vi "载荷控制.vi"() -> ()   [LabVIEW 2020]
doc: "The Basic Serial Read and Write example performs a Serial Port Read, a Serial Port Write, or a combination of these actions. The user selects the actions (read or write) on the front panel. If both are selected, the VI will write the data first, read data, and then close the VISA session that is opened to the port. This VI will wait until the specified number of bytes is received at the port. Only the number of bytes specified will be read.\n\nINSTRUCTIONS:\n1) Select the serial resource and configuration parameters (baud rate, data bits, parity, stop bits, flow control).\n2) Select the operations to be performed. \n3) Connect the serial port to your device. If no device is available, perform a loopback test by doing one of the following. Short pins 2 and 3 on a RS-232 cable or short pin 4 to pin 8 and pin 5 to pin 9 on a RS-485/422 cable. \n4) Run the VI to see the data read. (The \"read string\" will match the \"string to write\" if a loopback test was performed.)\n\nNote: The parameters set for the serial port must match the parameters of the connected instrument or device. In this example, the bytes to read parameter specifies the number of bytes that the serial port reads. If there were more bytes at the port than the number specified in bytes to read, those bytes would not be read. Also, if you specify to read more bytes than the number of bytes actually read, you might receive a timeout error message.\n\nOn the block diagram, the Configure Serial Port VI sets the configuration parameters. The front panel displays the controls used to configure the basic parameters, such as baud rate, data bits, and parity. Constants configure the other parameters the user probably does not need set. After the VISA Configure Serial Port VI opens the VISA session and configures the port, the VI passes the VISA resource name to other VIs that perform operations on that VISA resource. The VISA Write function sends a command to the serial device and the VISA Read function returns data based on the command. The VISA Close function then closes the reference to the serial device. It is important to close the reference; otherwise communication through with that port through protocols other than VISA might not be possible."
uses:
  <vilib>/Analysis/baseanly.llb/Mean (DBL).vi
  <vilib>/Instr/_visa.llb/VISA Configure Serial Port (Instr).vi
  <vilib>/addons/control/pid/pid.llb/PID (DBL).vi
  <vilib>/Analysis/NI_AALBase.lvlib
  <vilib>/addons/control/pid/NI_PID_pid.lvlib
panel:
  in  "点火/退出":bool
  in  "气缸":dbl
  in  "点火":dbl
  in  "停止3":bool
  out "位移(um）":dbl format="%#.2f"
  out "数据":dbl
  out "原始载荷":dbl format="%#.2f"
  out "当前次数":i32
  in  "选项卡控件":enum32{"设置", "手动", "自动", "循环加载"}(tab)
  in  "温度文件":path
  in  "设置串口":refnum<visa-resource-name>="COM1"
  in  "载荷测量":tag="cDAQ9184-1ADFF13Mod3"
  in  "气流控制":tag="Dev2"
  in  "?":bool
  in  "?":bool
  in  "?":bool
  in  "?":bool
  in  "位置清零":bool
  in  "载荷清零":bool
  in  "开始":bool
  in  "加载":bool
  in  "比例系数":i32 min=0 max=1000
  in  "设定载荷":i32 min=0 max=1000
  in  "形变速率（微米/秒）":i32 min=0
  in  "冷却控制":dbl
  in  "设定温度值 ℃":dbl(slide)=43.790849673202615 scale=0.0..3000.0
  out "MV：":dbl(slide)=18.78965245852964 scale=0.0..6.0
  in  "PID增益":T1={"比例增益(Kc)"=20.0, "积分时间（Ti，分）"=0.008, "微分时间（Td，分）"=0.001} {"微分时间（Td，分）" format="%.3f"; "积分时间（Ti，分）" format="%.3f"; "比例增益(Kc)" format="%.3f"}
  out "设定温度/实时温度 ℃":cluster{"initial PV":dbl, "SP:":dbl}(graph)
  in  "停止4":bool
  in  "喷火":dbl
  in  "开":bool
  in  "低载时间":dbl
  in  "高载时间":dbl
  in  "低载荷":dbl
  in  "高载荷":dbl
  in  "循环次数":i32
  out "载荷（N）":dbl format="%.2f"
  out "载荷零点\n（牛）":dbl
  in  "停止":bool
  out "拉压":dbl
  in  "触发":u8
  out "结果":i16
  in  "实际位置":i32
  out "位移(微米）":dbl
  in  "停止 2":bool
  in  "自动\n\n手动":bool
  # "微调"
  # "粗调"
  # "关"
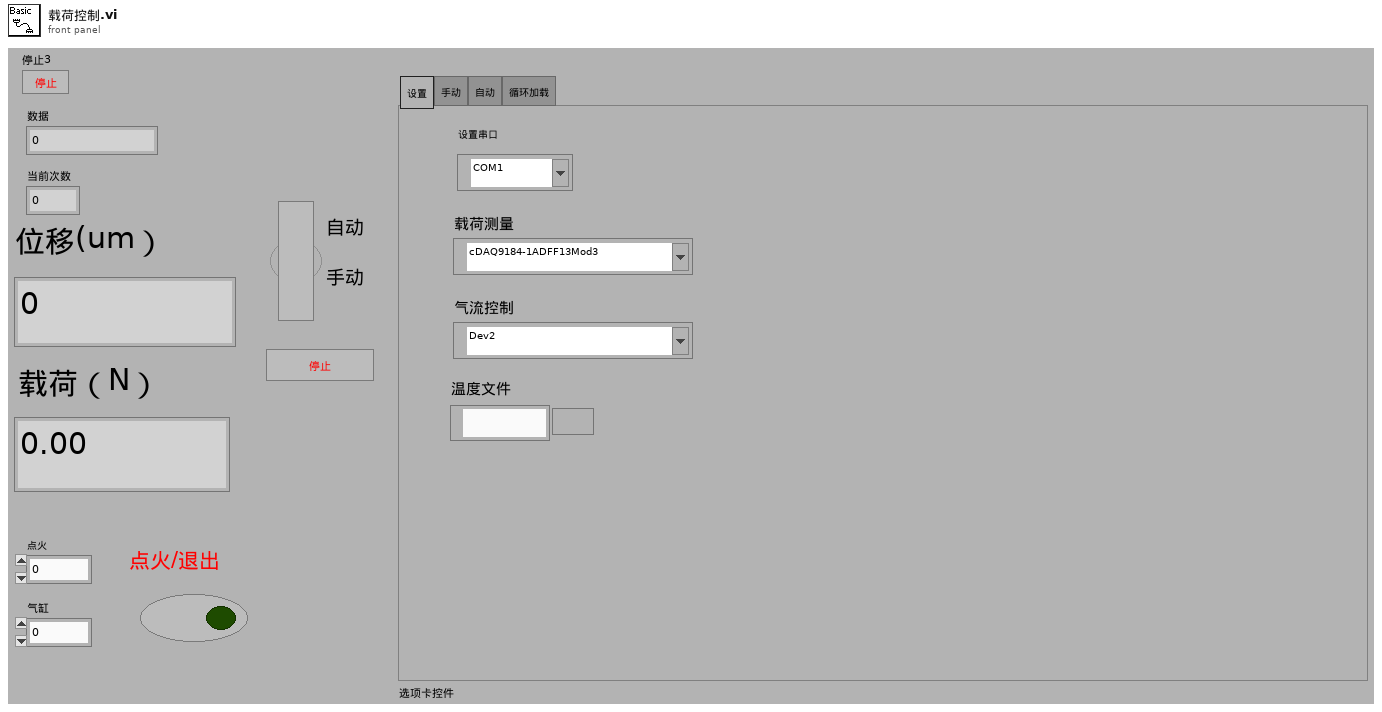
[diagram p1: front panel]
types:
  T1 = cluster{"比例增益(Kc)":dbl, "积分时间（Ti，分）":dbl, "微分时间（Td，分）":dbl}
  T2 = enum16{"open", "replace", "create", "open or create", "replace or create", "replace or create with confirmation"}
  T3 = cluster{"static gain":dbl, "lag (min)":dbl, "dead cycles":dbl, "load %":dbl, "deadband":dbl, "noise level %":dbl, "initial PV":dbl, "initial PV 2":dbl}
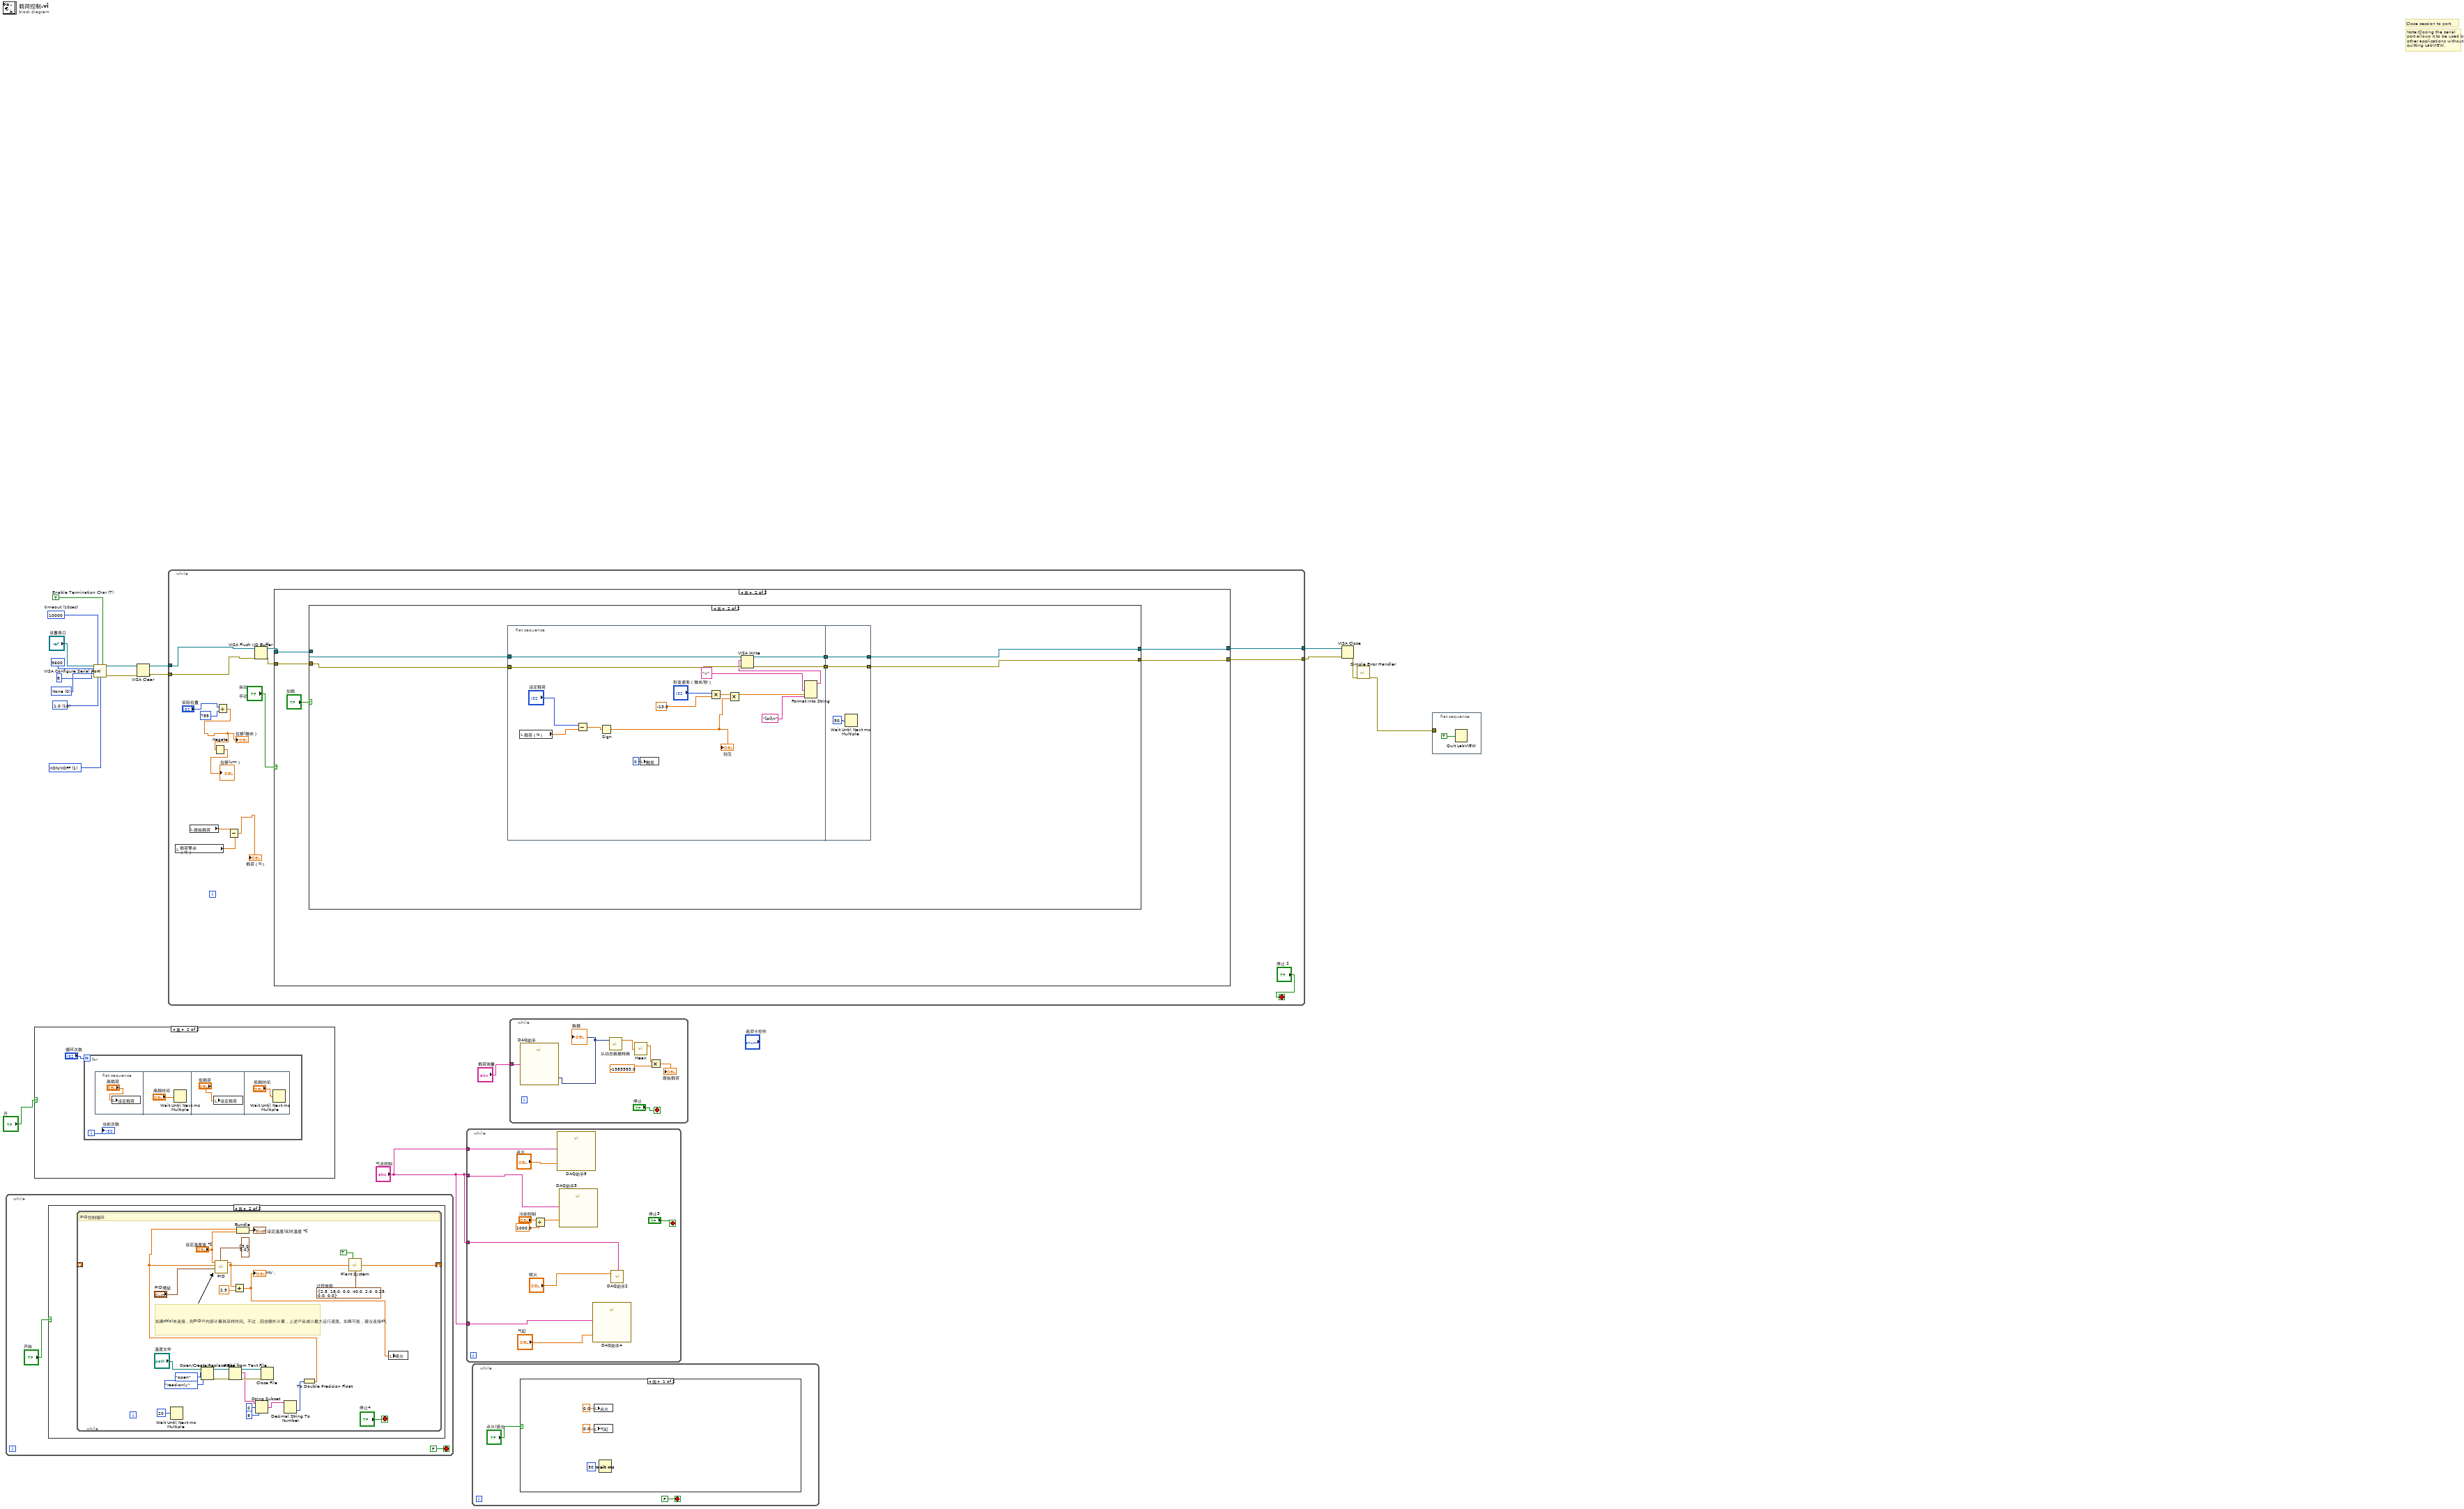
[diagram p0: block diagram]
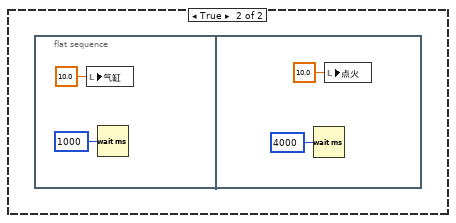
[diagram p2: hidden frame]
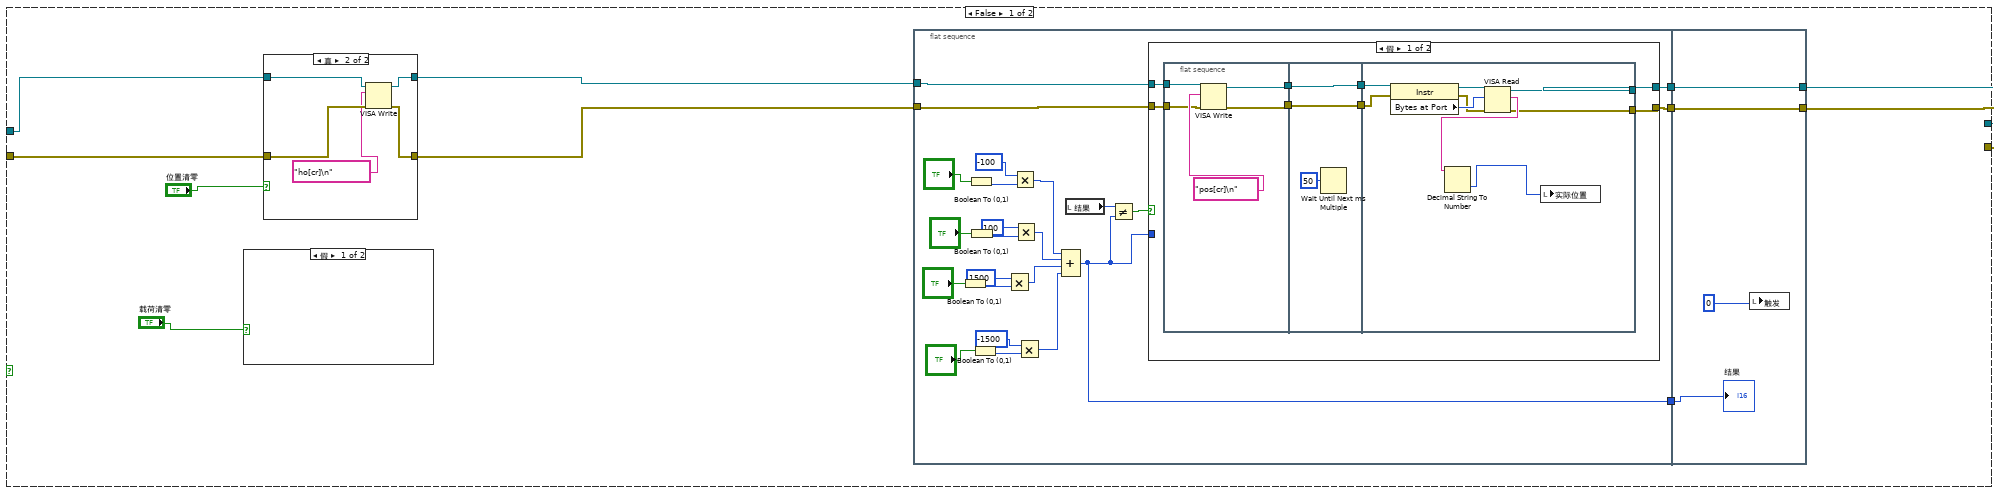
[diagram p5: hidden frame]
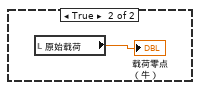
[diagram p6: hidden frame]
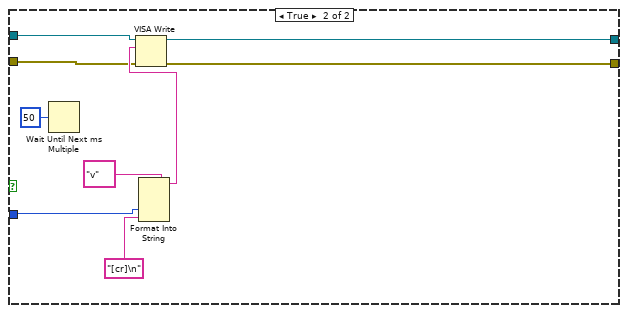
[diagram p8: hidden frame]
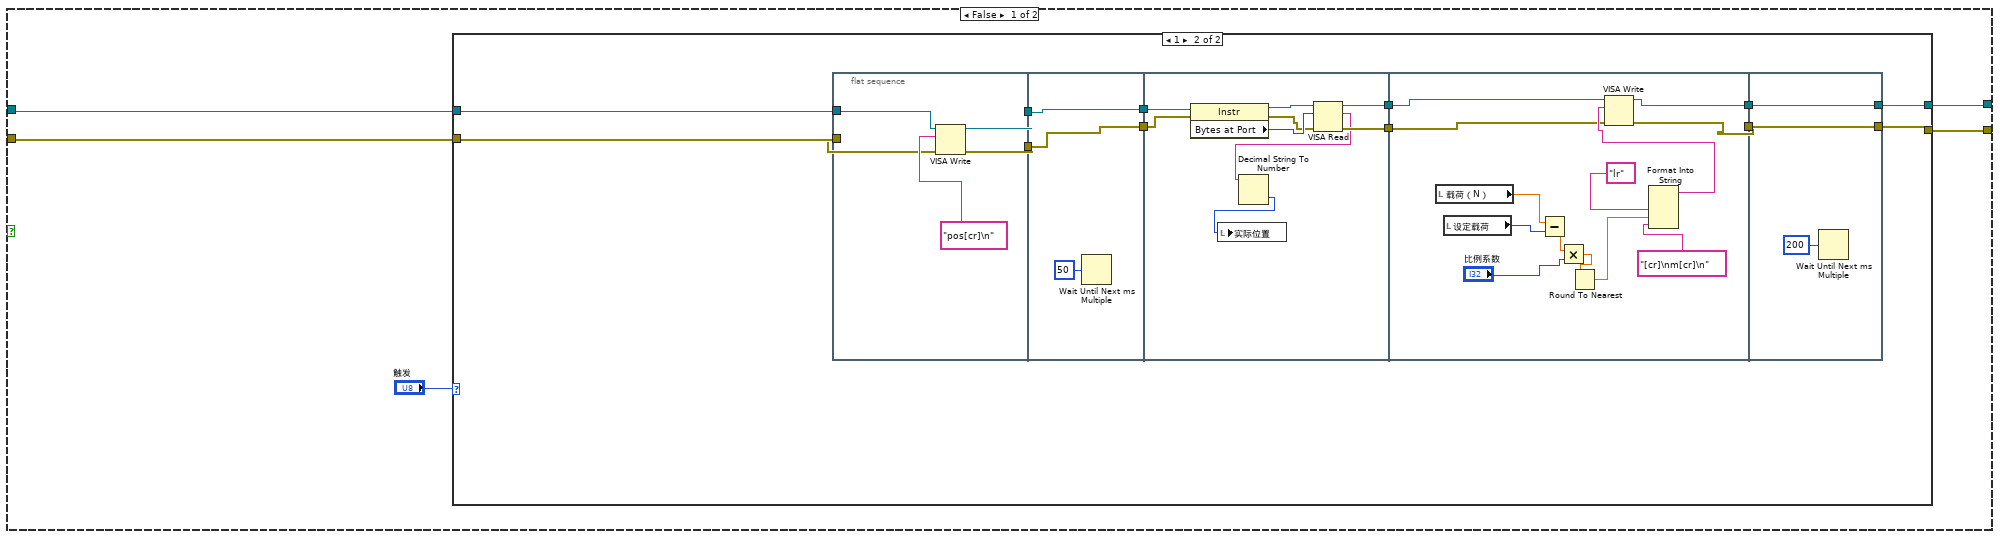
[diagram p9: hidden frame]
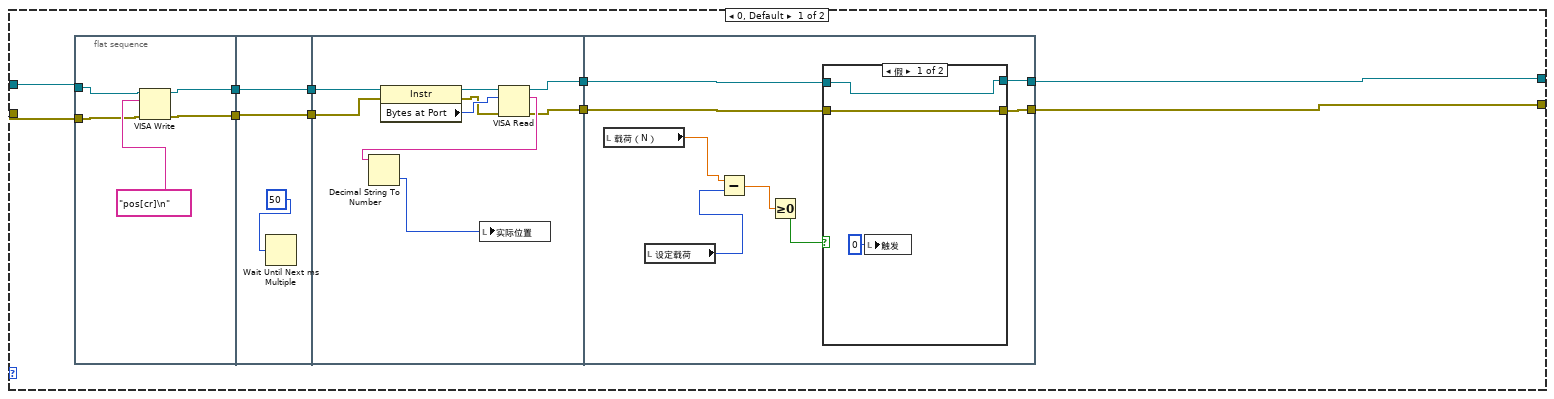
[diagram p10: hidden frame]
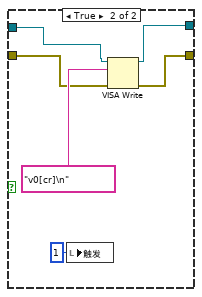
[diagram p11: hidden frame]
diagram:
  w13 = u16 1 items=["None"=0, "XON/XOFF"=1, "RTS/CTS"=2, "DTR/DSR"=4] ("flow control")
  w14 = u16 10 items=["1.0"=10, "1.5"=15, "2.0"=20] ("stop bits")
  w17 = u16 0 items=["None", "Odd", "Even", "Mark", "Space"] ("parity")
  w15 = TRUE  # Enable Termination Char (T)
  w16 = u32 10000  # timeout (10sec)
  # "Note:Closing the serial port allows it to be used by other applications without\nquitting LabVIEW."
  # "Close session to port."
  n1 = while {
    stop <- FALSE stop-if-true
    n2 = case shown="真" "开始" {
      frame False {
      }
      frame True {
        n3 = while {
          shift-left: _ -> [_]
          shift-right: [w23] -> _
          stop <- "停止4" stop-if-true
          w43 = T3 {"static gain"=2.5, "lag (min)"=18.0, "dead cycles"=0.0, "load %"=40.0, "deadband"=2.0, "noise level %"=0.25, "initial PV"=0.0, "initial PV 2"=0.0}  # 过程参数
          # "如果dt(s)未连接，则PIDVI内部计算其采样时间。不过，因含额外计算，上述VI会减小最大运行速度。如果可能，建议连接dt。"
          # "PID控制循环"
          n4 = Wait Until Next ms Multiple(millisecond multiple=u32 20 ("unsigned 32bit integer")) -> ()  [unwired: 1 out]
          n5 = Open/Create/Replace File(file path (use dialog)="温度文件", operation (0:open)=T2."open" ("操作(0:open)"), access (0:read/write)=enum16{"read/write", "read-only", "write-only"}."read-only" ("权限(0:read/write)")) -> (refnum out=w38:refnum<file>, error out=w40:errorcluster)  [unwired: 3 in, 1 out]
          n6 = Read from Text File(file (use dialog)=w38, error in=w40) -> (refnum out=w39:refnum<file>, text=w33:string, error out=w41:errorcluster)  [unwired: 2 in, 1 out]
          n7 = String Subset(string=w33, offset (0)=0 ("偏移量(0)"), length (rest)=8 ("长度（剩余）")) -> (substring=w30:string)
          n8 = Close File(refnum=w39, error in=w41) -> ()  [unwired: 2 out]
          n9 = Decimal String To Number(string=w30) -> (number=w29:i32)  [unwired: 2 in, 1 out]
          n10 = To Double Precision Float(number=w29) -> (double precision float=w31:dbl)
          n11 = call-poly <vilib>:"PID.vi"("output range"=cluster{"output high":dbl, "output low":dbl} {"output high"=3.0, "output low"=0.0}, "PID gains"="PID增益", "process variable"=w31, "setpoint"="设定温度值 ℃") -> ("output"=w27:dbl)  [unwired: 6 in, 1 out]
          n12 = Add(x=w27, y=2.5) -> (x+y=w22:dbl)
          "MV：" <- w22
          n13 = Bundle(w31, "设定温度值 ℃"="设定温度值 ℃") -> (→"设定温度/实时温度 ℃":cluster{dbl, "设定温度值 ℃":dbl})  [unwired: 1 in]
          n14 = call "Plant System.vi"("积分器？"=TRUE ("Integrator ?"), "设备输入"=w27, "过程参数"=w43) -> ("设备输出"=w23:dbl)  [unwired: 12 in]
          n15 = local write "喷火"(w22) -> ()
        }
      }
    }
  }
  n16 = case shown="真" "开" {
    frame False {
    }
    frame True {
      n17 = for {
        N: "循环次数" -> [_]
        i -> [w48]
        n18 = flat-sequence {
          frame #0 {
            n19 = local write "设定载荷"("高载荷") -> ()
          }
          frame #1 {
            n20 = Wait Until Next ms Multiple(millisecond multiple="高载时间") -> ()  [unwired: 1 out]
          }
          frame #2 {
            n21 = local write "设定载荷"("低载荷") -> ()
          }
          frame #3 {
            n22 = Wait Until Next ms Multiple(millisecond multiple="低载时间") -> ()  [unwired: 1 out]
          }
        }
        "当前次数" <- w48
      }
    }
  }
  n23 = call-poly "VISA Configure Serial Port"("VISA resource name"="设置串口", "timeout (10sec)"=w16, "Enable Termination\nChar (T)"=w15, "baud rate (9600)"=u32 9600 ("baud rate"), "data bits (8)"=u16 8 ("data bits"), "parity (0:none)"=w17, "stop bits (10: 1 bit)"=w14, "flow control (0:none)"=w13) -> ("VISA resource name out"=w5:refnum<visa-resource-name>, "error out"=w7:errorcluster)  [unwired: 6 in]
  n24 = VISA Clear(VISA resource name=w5, error in (no error)=w7) -> (VISA resource name out=w6:refnum<visa-resource-name>, error out=w8:errorcluster)
  n25 = while {
    tunnel: w6 -> [w58]
    tunnel: w8 -> [w59]
    tunnel: [w65] -> w10
    tunnel: [w64] -> w9
    stop <- "停止 2" stop-if-true
    n26 = local read "载荷零点\n（牛）"() -> (w56:dbl)
    n27 = local read "原始载荷"() -> (w57:dbl)
    n28 = Divide(x="实际位置", y=785) -> (x/y=w53:dbl)
    "位移(微米）" <- w53
    n29 = Negate(x=w53) -> (-x=→"位移(um）":dbl)
    n30 = Subtract(x=w57, y=w56) -> (x-y=→"载荷（N）":dbl)
    n31 = VISA Flush I/O Buffer(VISA resource name=w58, error in (no error)=w59) -> (VISA resource name out=w61:refnum<visa-resource-name>, error out=w60:errorcluster)  [unwired: 1 in]
    n32 = case shown="真" "自动\n\n手动" {
      tunnel: w61 -> [w73 w152]
      tunnel: w60 -> [w71 w148]
      tunnel: [w75 w150] -> w65
      tunnel: [w74 w149] -> w64
      frame False {
        n33 = case shown="假" "载荷清零" {
          frame False {
          }
          frame True {
            n34 = local read "原始载荷"() -> (→"载荷零点\n（牛）":dbl)
          }
        }
        n35 = case shown="真" "位置清零" {
          tunnel: w73 -> [w81 w86]
          tunnel: [w81 w85] -> w72
          tunnel: w71 -> [w80 w84]
          tunnel: [w80 w83] -> w70
          frame False {
          }
          frame True {
            n36 = VISA Write(VISA resource name=w86, write buffer="ho[cr]\n" ("输入 1"), error in (no error)=w84) -> (VISA resource name out=w85:refnum<visa-resource-name>, error out=w83:errorcluster)  [unwired: 1 out]
          }
        }
        n37 = flat-sequence {
          tunnel: [w109] -> w78
          tunnel: [w96] -> w76
          tunnel: [w95] -> w77
          tunnel: w72 -> [w92]
          tunnel: w70 -> [w93]
          tunnel: w78 -> [w146]
          tunnel: w77 -> [w147]
          tunnel: w76 -> [w145]
          tunnel: [w146] -> w75
          tunnel: [w145] -> w74
          frame #0 {
            n38 = Boolean To (0,1)(Boolean="?") -> (0, 1=w89:i16)
            n39 = Boolean To (0,1)(Boolean="?") -> (0, 1=w107:i16)
            n40 = Boolean To (0,1)(Boolean="?") -> (0, 1=w105:i16)
            n41 = Boolean To (0,1)(Boolean="?") -> (0, 1=w103:i16)
            n42 = Multiply(x=i16 1500, y=w89) -> (x*y=w87:i16)
            n43 = Multiply(x=i16 -100, y=w107) -> (x*y=w100:i16)
            n44 = Multiply(x=i16 100, y=w105) -> (x*y=w99:i16)
            n45 = Multiply(x=i16 -1500, y=w103) -> (x*y=w98:i16)
            n46 = Compound Arithmetic op=ADD(w100, w99, w87, w98) -> (w95:i16)
            n47 = local read "结果"() -> (w94:i16)
            n48 = Not Equal?(x=w94, y=w95) -> (x != y?=w97:bool)
            n49 = case shown="假" w97 {
              tunnel: w92 -> [w113 w137]
              tunnel: [w117 w140] -> w109
              tunnel: w95 -> [_ w139]
              tunnel: w93 -> [w112 w136]
              tunnel: [w114 w138] -> w96
              frame False {
                n50 = flat-sequence {
                  tunnel: [w119] -> w116
                  tunnel: [w118] -> w115
                  tunnel: w113 -> [w121]
                  tunnel: w112 -> [w120]
                  tunnel: w116 -> [w124]
                  tunnel: w115 -> [w123]
                  tunnel: [w124] -> w111
                  tunnel: [w123] -> w110
                  tunnel: [w131] -> w117
                  tunnel: [w129] -> w114
                  tunnel: w111 -> [w128]
                  tunnel: w110 -> [w127]
                  frame #0 {
                    n51 = VISA Write(VISA resource name=w121, write buffer="pos[cr]\n" ("输入 1"), error in (no error)=w120) -> (VISA resource name out=w119:refnum<visa-resource-name>, error out=w118:errorcluster)  [unwired: 1 out]
                  }
                  frame #1 {
                    n52 = Wait Until Next ms Multiple(millisecond multiple=u32 50 ("毫秒倍数")) -> ()  [unwired: 1 out]
                  }
                  frame #2 {
                    n53 = property class="Instr"(reference=w128, error in=w127) -> (reference out=w132:refnum<visa-resource-name>, error out=w130:errorcluster, "Bytes at Port"=w133:u32)
                    n54 = VISA Read(VISA resource name=w132, byte count=w133, error in (no error)=w130) -> (VISA resource name out=w131:refnum<visa-resource-name>, read buffer=w134:string, error out=w129:errorcluster)  [unwired: 1 out]
                    n55 = Decimal String To Number(string=w134) -> (number=w126:i32)  [unwired: 2 in, 1 out]
                    n56 = local write "实际位置"(w126) -> ()
                  }
                }
              }
              frame True {
                n57 = Wait Until Next ms Multiple(millisecond multiple=u32 50 ("毫秒倍数")) -> ()  [unwired: 1 out]
                n58 = Format Into String("v" ("输入 1"), w139, "[cr]\n" ("输入 3")) -> (resulting string=w141:string)  [unwired: 3 in, 1 out]
                n59 = VISA Write(VISA resource name=w137, write buffer=w141, error in (no error)=w136) -> (VISA resource name out=w140:refnum<visa-resource-name>, error out=w138:errorcluster)  [unwired: 1 out]
              }
            }
          }
          frame #1 {
            n60 = local write "触发"(u8 0 ("触发")) -> ()
            "结果" <- w147
          }
        }
      }
      frame True {
        n61 = case shown="真" "加载" {
          tunnel: w152 -> [w156 w252]
          tunnel: w148 -> [w155 w251]
          tunnel: [w154 w250] -> w150
          tunnel: [w157 w249] -> w149
          frame False {
            n62 = case shown="1" "触发" {
              tunnel: [w163 w206] -> w157
              tunnel: w156 -> [w162 w209]
              tunnel: w155 -> [w161 w208]
              tunnel: [w158 w207] -> w154
              frame 0, Default {
                n63 = flat-sequence {
                  tunnel: [w172] -> w167
                  tunnel: [w171] -> w166
                  tunnel: w161 -> [w168]
                  tunnel: w162 -> [w169]
                  tunnel: [w175] -> w165
                  tunnel: w167 -> [w175]
                  tunnel: [w174] -> w164
                  tunnel: w166 -> [w174]
                  tunnel: w165 -> [w184]
                  tunnel: w164 -> [w182]
                  tunnel: [w178] -> w160
                  tunnel: [w177] -> w159
                  tunnel: [w189] -> w158
                  tunnel: [w192] -> w163
                  tunnel: w160 -> [w191]
                  tunnel: w159 -> [w190]
                  frame #0 {
                    n64 = VISA Write(VISA resource name=w169, write buffer="pos[cr]\n" ("输入 1"), error in (no error)=w168) -> (VISA resource name out=w172:refnum<visa-resource-name>, error out=w171:errorcluster)  [unwired: 1 out]
                  }
                  frame #1 {
                    n65 = Wait Until Next ms Multiple(millisecond multiple=u32 50 ("等待时间（毫秒）")) -> ()  [unwired: 1 out]
                  }
                  frame #2 {
                    n66 = property class="Instr"(reference=w184, error in=w182) -> (reference out=w183:refnum<visa-resource-name>, error out=w179:errorcluster, "Bytes at Port"=w180:u32)
                    n67 = VISA Read(VISA resource name=w183, byte count=w180, error in (no error)=w179) -> (VISA resource name out=w177:refnum<visa-resource-name>, read buffer=w181:string, error out=w178:errorcluster)  [unwired: 1 out]
                    n68 = Decimal String To Number(string=w181) -> (number=w176:i32)  [unwired: 2 in, 1 out]
                    n69 = local write "实际位置"(w176) -> ()
                  }
                  frame #3 {
                    n70 = local read "载荷（N）"() -> (w186:dbl)
                    n71 = local read "设定载荷"() -> (w188:i32)
                    n72 = Subtract(x=w186, y=w188) -> (x-y=w185:dbl)
                    n73 = Greater Or Equal To 0?(x=w185) -> (x >= 0?=w187:bool)
                    n74 = case shown="假" w187 {
                      tunnel: [w194 w199] -> w192
                      tunnel: [w193 w198] -> w189
                      tunnel: w191 -> [w194 w196]
                      tunnel: w190 -> [w193 w197]
                      frame False {
                        n75 = local write "触发"(u8 0 ("触发")) -> ()
                      }
                      frame True {
                        n76 = local write "触发"(u8 1 ("触发")) -> ()
                        n77 = VISA Write(VISA resource name=w197, write buffer="v0[cr]\n" ("输入 1"), error in (no error)=w196) -> (VISA resource name out=w198:refnum<visa-resource-name>, error out=w199:errorcluster)  [unwired: 1 out]
                      }
                    }
                  }
                }
              }
              frame 1 {
                n78 = flat-sequence {
                  tunnel: [w217] -> w212
                  tunnel: [w216] -> w210
                  tunnel: w208 -> [w215]
                  tunnel: w209 -> [w214]
                  tunnel: [w221] -> w213
                  tunnel: w212 -> [w221]
                  tunnel: [w220] -> w211
                  tunnel: w210 -> [w220]
                  tunnel: w211 -> [w223]
                  tunnel: w213 -> [w224]
                  tunnel: [w230] -> w205
                  tunnel: [w229] -> w204
                  tunnel: [w240] -> w203
                  tunnel: [w241] -> w202
                  tunnel: w204 -> [w238]
                  tunnel: w205 -> [w237]
                  tunnel: [w245] -> w206
                  tunnel: [w246] -> w207
                  tunnel: w203 -> [w246]
                  tunnel: w202 -> [w245]
                  frame #0 {
                    n79 = VISA Write(VISA resource name=w214, write buffer="pos[cr]\n" ("输入 1"), error in (no error)=w215) -> (VISA resource name out=w217:refnum<visa-resource-name>, error out=w216:errorcluster)  [unwired: 1 out]
                  }
                  frame #1 {
                    n80 = Wait Until Next ms Multiple(millisecond multiple=u32 50 ("毫秒倍数")) -> ()  [unwired: 1 out]
                  }
                  frame #2 {
                    n81 = property class="Instr"(reference=w224, error in=w223) -> (reference out=w228:refnum<visa-resource-name>, error out=w225:errorcluster, "Bytes at Port"=w226:u32)
                    n82 = VISA Read(VISA resource name=w228, byte count=w226, error in (no error)=w225) -> (VISA resource name out=w230:refnum<visa-resource-name>, read buffer=w227:string, error out=w229:errorcluster)  [unwired: 1 out]
                    n83 = Decimal String To Number(string=w227) -> (number=w222:i32)  [unwired: 2 in, 1 out]
                    n84 = local write "实际位置"(w222) -> ()
                  }
                  frame #3 {
                    n85 = local read "载荷（N）"() -> (w236:dbl)
                    n86 = local read "设定载荷"() -> (w235:i32)
                    n87 = Subtract(x=w236, y=w235) -> (x-y=w234:dbl)
                    n88 = Multiply(x=w234, y="比例系数") -> (x*y=w232:dbl)
                    n89 = Round To Nearest(number=w232) -> (nearest integer value=w231:dbl)
                    n90 = Format Into String("lr" ("输入 1"), w231, "[cr]\nm[cr]\n" ("输入 3")) -> (resulting string=w239:string)  [unwired: 3 in, 1 out]
                    n91 = VISA Write(VISA resource name=w237, write buffer=w239, error in (no error)=w238) -> (VISA resource name out=w240:refnum<visa-resource-name>, error out=w241:errorcluster)  [unwired: 1 out]
                  }
                  frame #4 {
                    n92 = Wait Until Next ms Multiple(millisecond multiple=u32 200 ("毫秒倍数")) -> ()  [unwired: 1 out]
                  }
                }
              }
            }
          }
          frame True {
            n93 = flat-sequence {
              tunnel: w252 -> [w268]
              tunnel: w251 -> [w267]
              tunnel: [w266] -> w248
              tunnel: [w265] -> w247
              tunnel: [w270] -> w249
              tunnel: [w271] -> w250
              tunnel: w248 -> [w271]
              tunnel: w247 -> [w270]
              frame #0 {
                n94 = local read "载荷（N）"() -> (w256:dbl)
                n95 = Subtract(x="设定载荷", y=w256) -> (x-y=w255:dbl)
                n96 = Sign(1:w255) -> (0:w253:dbl)
                "拉压" <- w253
                n97 = local write "触发"(u8 0 ("触发")) -> ()
                n98 = Multiply(x="形变速率（微米/秒）", y=-13.0 ("x")) -> (x*y=w260:dbl)
                n99 = Multiply(x=w260, y=w253) -> (x*y=w254:dbl)
                n100 = Format Into String("v" ("输入 1"), w254, "[cr]\n" ("输入 3")) -> (resulting string=w262:string)  [unwired: 3 in, 1 out]
                n101 = VISA Write(VISA resource name=w268, write buffer=w262, error in (no error)=w267) -> (VISA resource name out=w266:refnum<visa-resource-name>, error out=w265:errorcluster)  [unwired: 1 out]
              }
              frame #1 {
                n102 = Wait Until Next ms Multiple(millisecond multiple=u32 50 ("毫秒倍数")) -> ()  [unwired: 1 out]
              }
            }
          }
        }
      }
    }
  }
  n103 = while {
    tunnel: "气流控制" -> [w282]
    tunnel: "气流控制" -> [w276]
    tunnel: "气流控制" -> [w274]
    tunnel: "气流控制" -> [w273]
    stop <- "停止3" stop-if-true
    n104 = Divide(x="冷却控制", y=1000.0) -> (x/y=w279:dbl)
    n105 = call "DAQ助手5"("data"="点火", "设备名"=w276) -> ()  [unwired: 16 in, 2 out]
    n106 = call "DAQ助手3"("data"=w279, "设备名"=w282) -> ()  [unwired: 16 in, 2 out]
    n107 = call "DAQ助手4"("data"="气缸", "设备名"=w273) -> ()  [unwired: 16 in, 2 out]
    n108 = call "DAQ助手2"("data"="喷火", "设备名"=w274) -> ()  [unwired: 16 in, 2 out]
  }
  n109 = while {
    stop <- FALSE stop-if-true
    n110 = case shown="假" "点火/退出" {
      frame False {
        n111 = local write "点火"(0.0 ("点火")) -> ()
        n112 = local write "气缸"(0.0 ("气缸")) -> ()
        n113 = Wait (ms)(milliseconds to wait=u32 30 ("等待时间（毫秒）")) -> ()  [unwired: 1 out]
      }
      frame True {
        n114 = flat-sequence {
          frame #0 {
            n115 = local write "气缸"(10.0 ("气缸")) -> ()
            n116 = Wait (ms)(milliseconds to wait=u32 1000 ("等待时间（毫秒）")) -> ()  [unwired: 1 out]
          }
          frame #1 {
            n117 = Wait (ms)(milliseconds to wait=u32 4000 ("等待时间（毫秒）")) -> ()  [unwired: 1 out]
            n118 = local write "点火"(10.0 ("点火")) -> ()
          }
        }
      }
    }
  }
  n119 = while {
    tunnel: "载荷测量" -> [w292]
    stop <- "停止" stop-if-true
    n120 = call "DAQ助手"("设备名"=w292) -> ("data"=w294:dynamicdata)  [unwired: 16 in, 2 out]
    "数据" <- w294
    n121 = call "从动态数据转换"("Dynamic Data Type"=w294) -> ("Array"=w295:dbl[])  [unwired: 3 in]
    n122 = call-poly <vilib>:"Mean.vi"("X"=w295) -> ("mean"=w293:dbl)  [unwired: 1 out]
    n123 = Multiply(x=w293, y=-1383583.0) -> (x*y=→"原始载荷":dbl)
  }
  n124 = VISA Close(VISA resource name=w10, error in (no error)=w9) -> (error out=w18:errorcluster)
  n125 = call <vilib>:"Simple Error Handler.vi"("error in (no error)"=w18) -> ("error out"=w4:errorcluster)  [unwired: 4 in, 4 out]
  n126 = flat-sequence {
    tunnel: w4 -> [_]
    frame #0 {
      n127 = Quit LabVIEW(quit? (T)=TRUE ("退出？(T)")) -> ()
    }
  }
